vi "Automotive ECU - Fault Control.vi"() -> ()   [LabVIEW 2013]
doc: "Sample numeric display item."
uses:
  <vilib>/NI Veristand/Display Template Support/Display Template Support.llb/cluster_Screen Item Settings.ctl
  <vilib>/NI Veristand/Display Template Support/Display Template Support.llb/cluster_Graph Scale Settings.ctl
  <vilib>/NI Veristand/Display Template Support/Display Template Support.llb/cluster_Graph Plot Settings.ctl
  NationalInstruments.VeriStand.SystemStorage
  Support/Fault Control.ctl
  <vilib>/NI Veristand/Display Template Support/Display Template Support.llb/enum_Display Template Handler Minimal To Widget Msg.ctl
  <vilib>/NI Veristand/Display Template Support/Display Template Support.llb/enum_Display Template Handler Minimal To Workspace.ctl
  Support/Fault Control Parameters.ctl
  <vilib>/NI Veristand/Execution/Workspace/NI VeriStand - Set Single Channel Value.vi
  <vilib>/NI Veristand/Execution/Workspace/NI_VS Workspace ExecutionAPI.lvlib
panel:
  in  "Multi- Lock":bool
  in  "Array":T1=[{"String"="Display Name \n", "String 2"="", "String 3"="", "Radio Buttons"=enum."Radio Selection 1"}]
  out "Label":string="Numeric"
  in  "NIVS.System Definition Root":refnum<k24>
  in  "NIVS.Gateway IP Address":string
  in  "Item.Data":T2
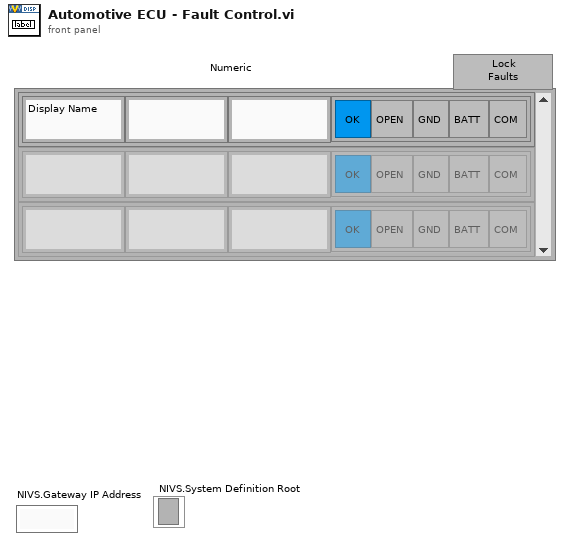
[diagram p1: front panel]
types:
  T1 = typedef "Fault Control.ctl" = cluster{"String":string, "String 2":string, "String 3":string, "Radio Buttons":enum32{"Radio Selection 1", "Radio Selection 2", "Radio Selection 3", "Radio Selection 4", "Radio Selection 5"}}[]
  T2 = typedef "cluster_Screen Item Settings.ctl" = cluster{"Template VI":string, "Position X":i32, "Position Y":i32, "Custom":string, "Show Title Bar":bool, "ID":i32, "Always On Top":bool, "Allow Resize":bool, "Allow Minimize":bool, "Allow Close":bool, "Size to Screen":bool, "Screen.ID":i32, "State":enum16{"Normal", "New"}, "Title":string, "Window Bounds":cluster{"[0]":i16, "[1]":i16, "[2]":i16, "[3]":i16}, "Channel Ref":u64, "Unit":string, "Default Units?":bool, "Flash Limit?":bool, "Color 1":u32, "Color 2":u32, "Color 3":u32, "Color 4":u32, "Bck Color":u32, "Fore Color":u32, "Limit 1":dbl, "Limit 2":dbl, "Limit 3":dbl, "Limit 4":dbl, "Limit Mode 1":i32, "Limit Mode 2":i32, "Limit Mode 3":i32, "Limit Mode 4":i32, "Scale Precision":i32, "Scale Min":dbl, "Scale Max":dbl, "Format":i32, "Precision":i32, "Background Type":i32, "IDs":i32[], "Units":string[], "Labels":string[], "Scale Factor":dbl, "Scale Offset":dbl, "YScale Index":u32[], "XScale":T3, "YScales":T3[], "Plots":T4[], "Update Period":dbl, "History Length":dbl, "My.Ref":refnum<vi>, "Is Control?":bool, "Channel Paths":string[], "Custom Data":variant}
  T3 = typedef "cluster_Graph Scale Settings.ctl" = cluster{"Format":u8, "Precision":u8, "Fit":u8, "Label":string, "Use Default Label":bool, "Label Visible":bool, "Min":dbl, "Max":dbl}
  T4 = typedef "cluster_Graph Plot Settings.ctl" = cluster{"Bar Style":u8, "Fill To":i16, "Fill/PtColor":u32, "Line Style":u8, "Line Width":u8, "Color":u32, "Interp":u8, "Point Style":u8}
  T5 = typedef "enum_Display Template Handler Minimal To Workspace.ctl" = cluster{"Operation":enum16{"SetCustomData", "DeleteItem"}, "Data":variant}
  T6 = typedef "enum_Display Template Handler Minimal To Widget Msg.ctl" = enum16{"Stop", "LaunchConfigDialog"}
  T7 = typedef "Fault Control Parameters.ctl" = cluster{"Initialized?":bool, "Label":string, "Default Control Values":variant[], "Channel Array":cluster{"NodePathArray":string[], "Node Path":string}[], "Fault Control":cluster{"String":string, "String 2":string, "String 3":string, "Radio Buttons":enum32{"Radio Selection 1", "Radio Selection 2", "Radio Selection 3", "Radio Selection 4", "Radio Selection 5"}}[], "Signals out Array":dbl[]}
  T8 = typedef "NI_VS Workspace ExecutionAPI.lvlib/WorkspaceAPI.ctl" = refnum<k24>
  T9 = cluster{"NodePathArray":string[], "Node Path":string}[]
  T10 = enum32{"Radio Selection 1", "Radio Selection 2", "Radio Selection 3", "Radio Selection 4", "Radio Selection 5"}
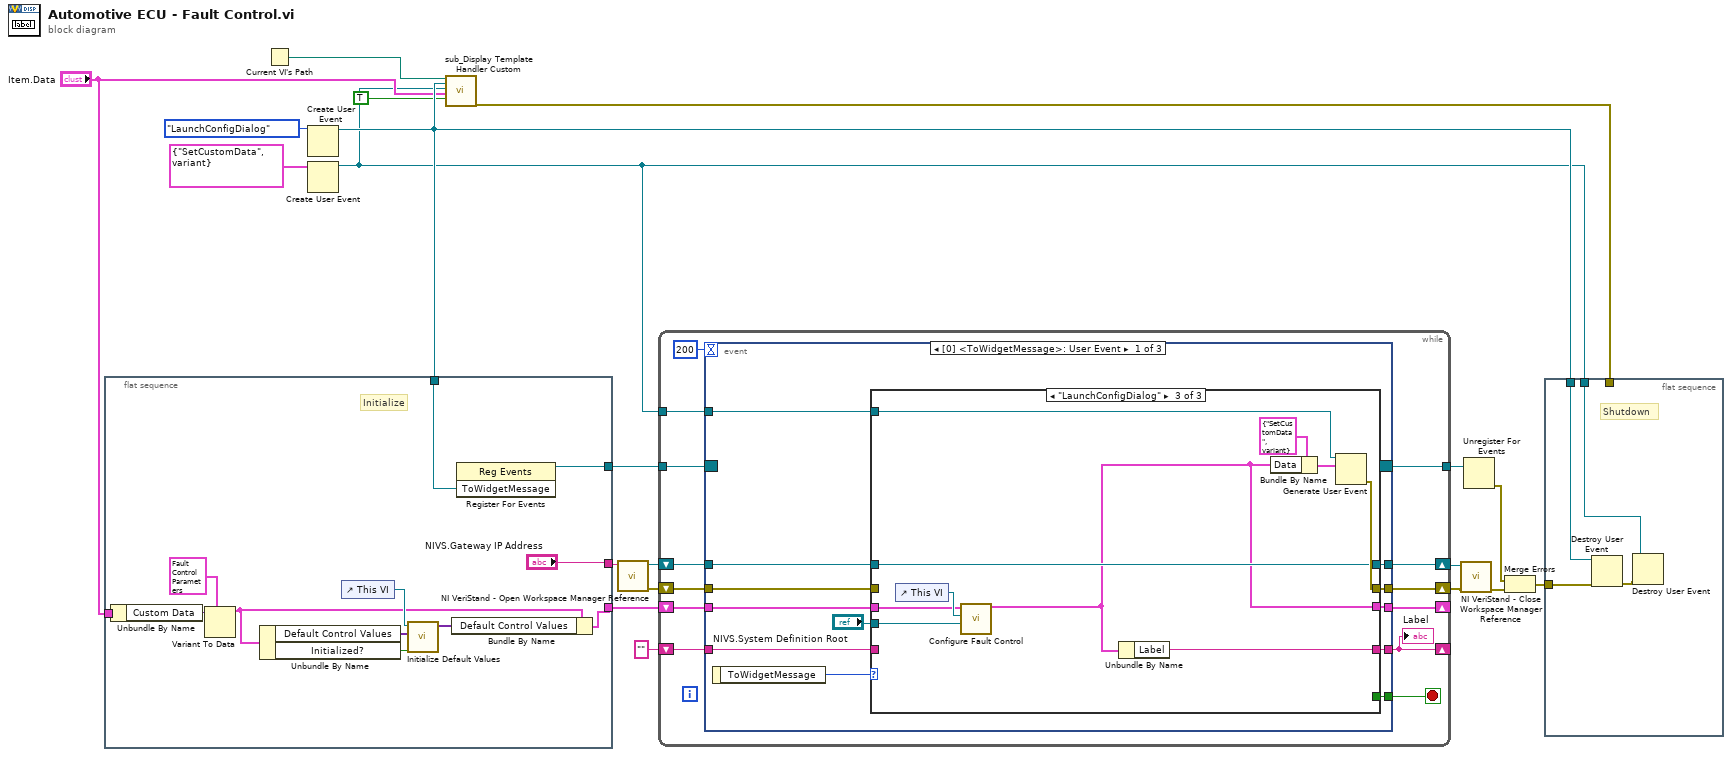
[diagram p0: block diagram]
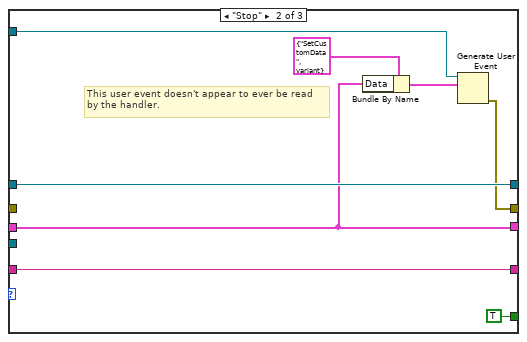
[diagram p3: hidden frame]
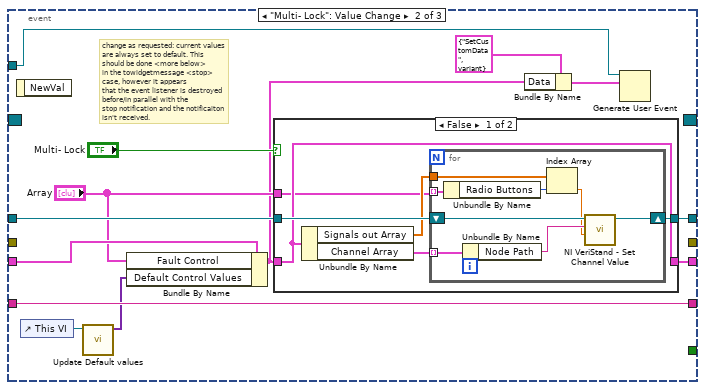
[diagram p4: hidden frame]
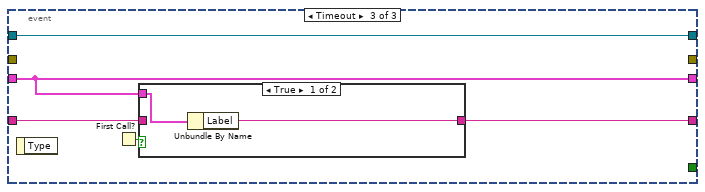
[diagram p6: hidden frame]
diagram:
  n1 = flat-sequence {
    tunnel: [w32] -> w18
    tunnel: w15 -> [w31]
    tunnel: "Item.Data" -> [w30]
    tunnel: [w23] -> w9
    tunnel: ["NIVS.Gateway IP Address"] -> w6
    frame #0 {
      # "Initialize"
      n2 = Unbundle By Name(w30) -> ("Custom Data"=w29:variant)
      n3 = Variant To Data(type=T7 {"Initialized?"=FALSE, "Label"="", "Default Control Values"=[], "Channel Array"=[], "Fault Control"=[{"String"="", "String 2"="", "String 3"="", "Radio Buttons"=enum."Radio Selection 1"}, {"String"="", "String 2"="", "String 3"="", "Radio Buttons"=enum."Radio Selection 1"}, {"String"="", "String 2"="", "String 3"="", "Radio Buttons"=enum."Radio Selection 1"}, {"String"="", "String 2"="", "String 3"="", "Radio Buttons"=enum."Radio Selection 1"}], "Signals out Array"=[]} ("Slide Parameters"), Variant=w29) -> (data=w22:T7)  [unwired: 1 in, 1 out]
      n4 = Unbundle By Name(w22) -> ("Default Control Values"=w26:variant[], "Initialized?"=w24:bool)
      n5 = control-ref of="This VI"() -> (w25:refnum<vi>)
      n6 = call "Initialize Default Values.vi"("Initialized?"=w24, "Default Control Values in"=w26, "VI in"=w25) -> ("Default Control Values out"=w27:variant[])  [unwired: 7 in, 1 out]
      n7 = Bundle By Name(cluster=w22, "Default Control Values"=w27) -> (w23:T7)
      n8 = register-events(w31) -> (reference out=w32:refnum<event-registration>)  [unwired: 2 in, 1 out]
    }
  }
  n9 = Current VI's Path() -> (path=w13:path)
  n10 = Create User Event(user event datatype=enum_Display_Template_Handler_Minimal_To_Widget_Msg."LaunchConfigDialog" ("ToWidgetMessage")) -> (user event=w15:refnum<user-event>)  [unwired: 1 in, 1 out]
  n11 = Create User Event(user event datatype=T5 {"Operation"=enum."SetCustomData", "Data"=variant} ("Data")) -> (user event=w11:refnum<user-event>)  [unwired: 1 in, 1 out]
  n12 = call <vilib>:"sub_Display Template Handler Custom.vi"("Parent.Path"=w13, "ToWidgetEvent"=w15, "ToWorkspace"=w11, "Item.Data"="Item.Data", "Resizable"=TRUE) -> ("error out"=w20:errorcluster)  [unwired: 14 in]
  n13 = call <vilib>:"NI VeriStand - Open Workspace Manager Reference.vi"("Gateway IP Address (\"\": localhost)"=w6) -> ("error out"=w7:errorcluster, "WorkspaceManager"=w8:T8)  [unwired: 9 in]
  n14 = while {
    tunnel: w18 -> [w45]
    tunnel: [w43] -> w17
    tunnel: w11 -> [w42]
    shift-right: [w34] -> _
    shift-left: w9 -> [w41]
    shift-right: [w38] -> w3
    shift-left: w8 -> [w40]
    shift-right: [w35] -> w2
    shift-left: w7 -> [w39]
    shift-right: [w36] -> _
    shift-left: "" ("Out") -> [w37]
    stop <- w44 stop-if-true
    n15 = event shown="[0] <ToWidgetMessage>: User Event" {
      selector: w45 -> [_ _ _]
      dyn-events: [_ _ _] -> w43
      timeout: 200 -> [_ _ _]
      tunnel: [w56 _ _] -> w44
      tunnel: w42 -> [w55 w81 _]
      tunnel: w41 -> [w51 w87 w110]
      tunnel: w40 -> [w54 w90 w109]
      tunnel: w39 -> [w49 _ _]
      tunnel: [w53 w89 w109] -> w38
      tunnel: [w48 _ _] -> w35
      tunnel: [w47 w92 w112] -> w36
      tunnel: w37 -> [w46 w92 w111]
      tunnel: [w50 w88 w110] -> w34
      event User Event {
        n16 = event-data() -> ("ToWidgetMessage"=w57:T6)  [unwired: 1 out]
        n17 = case shown="\"LaunchConfigDialog\"" w57 {
          tunnel: [_ TRUE _] -> w56
          tunnel: w55 -> [_ w65 w77]
          tunnel: w54 -> [w61 w68 w72]
          tunnel: [w61 w68 w72] -> w53
          tunnel: "NIVS.System Definition Root" -> [_ _ w75]
          tunnel: w51 -> [w60 w62 w70]
          tunnel: [w60 w62 w71] -> w50
          tunnel: w49 -> [w58 _ _]
          tunnel: [w58 w64 w76] -> w48
          tunnel: [w59 w63 w73] -> w47
          tunnel: w46 -> [w59 w63 _]
          frame Default {
          }
          frame "Stop" {
            # "This user event doesn't appear to ever be read\nby the handler."
            n18 = Bundle By Name(cluster=T5 {"Operation"=enum."SetCustomData", "Data"=variant} ("event data"), "Data"=w62) -> (w66:T5)
            n19 = Generate User Event(user event=w65, event data cluster=w66) -> (error out=w64:errorcluster)  [unwired: 2 in, 1 out]
          }
          frame "LaunchConfigDialog" {
            n20 = control-ref of="This VI"() -> (w74:refnum<vi>)
            n21 = call "Configure Fault Control.vi"("NIVS.System Definition Root"=w75, "VI Reference"=w74, "Fault Parameters in"=w70) -> ("Fault Parameters out"=w71:T7)  [unwired: 7 in, 1 out]
            n22 = Unbundle By Name(w71) -> ("Label"=w73:string)
            n23 = Bundle By Name(cluster=T5 {"Operation"=enum."SetCustomData", "Data"=variant} ("event data"), "Data"=w71) -> (w79:T5)
            n24 = Generate User Event(user event=w77, event data cluster=w79) -> (error out=w76:errorcluster)  [unwired: 2 in, 1 out]
          }
        }
      }
      event "Multi- Lock": Value Change {
        # "change as requested: current values\nare always set to default. This should be done <more below>\nin the towidgetmessage <stop> case, however it appears\nthat the event listener is destroyed before/in parallel with the\nstop notification and the notificaiton isn't received."
        n25 = event-data() -> ()  [unwired: 2 out]
        n26 = control-ref of="This VI"() -> (w85:refnum<vi>)
        n27 = call "Update Default values.vi"("VI in"=w85) -> ("Default Values out"=w84:variant[])  [unwired: 10 in]
        n28 = Bundle By Name(cluster=w87, "Fault Control"="Array", "Default Control Values"=w84) -> (w80:T7)
        n29 = case shown="False" "Multi- Lock" {
          tunnel: w80 -> [w94 w108]
          tunnel: w90 -> [w97 w107]
          tunnel: [w95 w107] -> w89
          tunnel: [w94 w108] -> w88
          tunnel: "Array" -> [w93 _]
          frame False {
            n30 = Unbundle By Name(w94) -> ("Signals out Array"=w96:dbl[], "Channel Array"=w98:T9)
            n31 = for {
              tunnel: w93 -> [w106] mode=indexing
              tunnel: w98 -> [w104] mode=indexing
              tunnel: w96 -> [w100]
              shift-right: [w99] -> w95
              shift-left: w97 -> [w103]
              n32 = Unbundle By Name(w106) -> ("Radio Buttons"=w105:T10)
              n33 = Unbundle By Name(w104) -> ("Node Path"=w102:string)
              n34 = Index Array(array=w100, index=w105) -> (element=w101:dbl)
              n35 = call-poly <vilib>:"NI VeriStand - Set Channel Value.vi"("Value"=w101, "Channel"=w102, "WorkspaceManager in"=w103) -> ("WorkspaceManager out"=w99:T8)  [unwired: 7 in, 1 out]
            }
          }
          frame True {
          }
        }
        n36 = Bundle By Name(cluster=T5 {"Operation"=enum."SetCustomData", "Data"=variant} ("event data"), "Data"=w80) -> (w82:T5)
        n37 = Generate User Event(user event=w81, event data cluster=w82) -> ()  [unwired: 2 in, 2 out]
      }
      event Timeout {
        n38 = event-data() -> ()  [unwired: 2 out]
        n39 = First Call?() -> (First Call?: T/F=w113:bool)
        n40 = case shown="True" w113 {
          tunnel: w111 -> [_ w116]
          tunnel: [w114 w116] -> w112
          tunnel: w110 -> [w115 _]
          frame True {
            n41 = Unbundle By Name(w115) -> ("Label"=w114:string)
          }
          frame False {
            # "If this is the first call, update label"
          }
        }
      }
    }
    "Label" <- w36
  }
  n42 = call <vilib>:"NI VeriStand - Close Workspace Manager Reference.vi"("error in (no error)"=w2, "WorkspaceManager"=w3) -> ("error out"=w1:errorcluster)  [unwired: 9 in]
  n43 = Unregister For Events(event registration refnum=w17) -> (error out=w16:errorcluster)  [unwired: 1 in]
  n44 = Merge Errors(w16, w1) -> (w4:errorcluster)
  n45 = flat-sequence {
    tunnel: w20 -> [_]
    tunnel: w15 -> [w120]
    tunnel: w11 -> [w118]
    tunnel: w4 -> [w117]
    frame #0 {
      # "Shutdown"
      n46 = Destroy User Event(user event=w120, error in=w117) -> (error out=w119:errorcluster)
      n47 = Destroy User Event(user event=w118, error in=w119) -> ()  [unwired: 1 out]
    }
  }
